vi "p_edge.vi"(11 "In":bool) -> (3 "Out":bool)   [LabVIEW 2013]
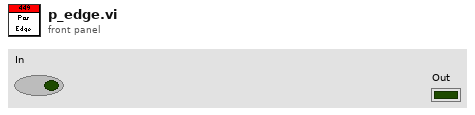
[diagram p1: front panel]
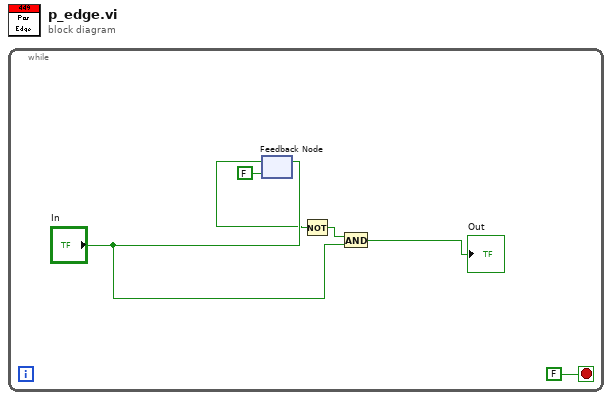
[diagram p0: block diagram]
diagram:
  n1 = while {
    stop <- FALSE stop-if-true
    n2 = feedback #1(FALSE ("In")) -> (w3:bool)
    n3 = feedback-in #1("In") -> ()
    n4 = Not(x=w3) -> (.not. x?=w4:bool)
    n5 = And(x=w4, y="In") -> (x .and. y?=→"Out":bool)
  }
